vi "Main.vi"() -> ()   [LabVIEW 2017]
uses:
  Controls/SM_Control.ctl
  Controls/Operaciones.ctl
panel:
  in  "ON/OFF":bool
  in  "Clear":bool
  out "Display":string
  in  "Teclas":T1
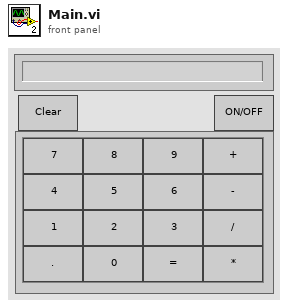
[diagram p1: front panel]
types:
  T1 = cluster{"Cero":bool, "Uno":bool, "Dos":bool, "Tres":bool, "Cuatro":bool, "Cinco":bool, "Seis":bool, "Siete":bool, "Ocho":bool, "Nueve":bool, "Punto":bool, "Igual":bool, "Mas":bool, "Resta":bool, "Div":bool, "Multp":bool}
  T2 = typedef "SM_Control.ctl" = enum16{"Inicializar", "Event Handler", "Tecla", "Stop", "Clear", "ON/OFF"}
  T3 = typedef "Operaciones.ctl" = enum16{"Suma", "Resta", "Mult", "Div"}
  T4 = enum8{"Enabled", "Disabled", "Disabled and Grayed Out"}
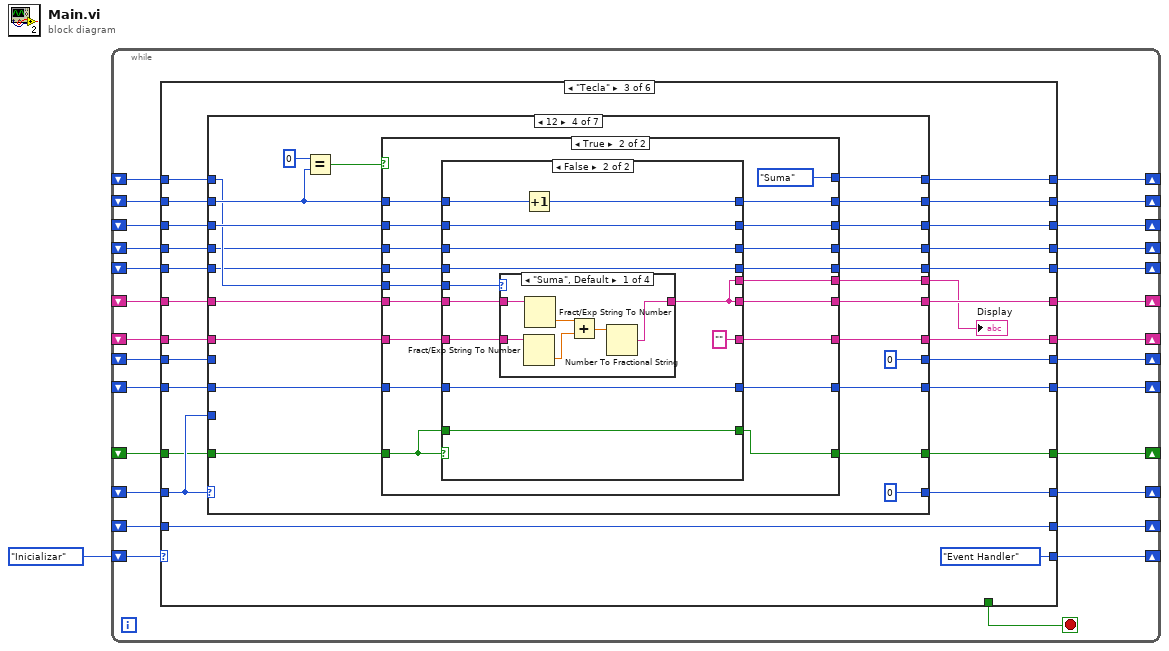
[diagram p0: block diagram]
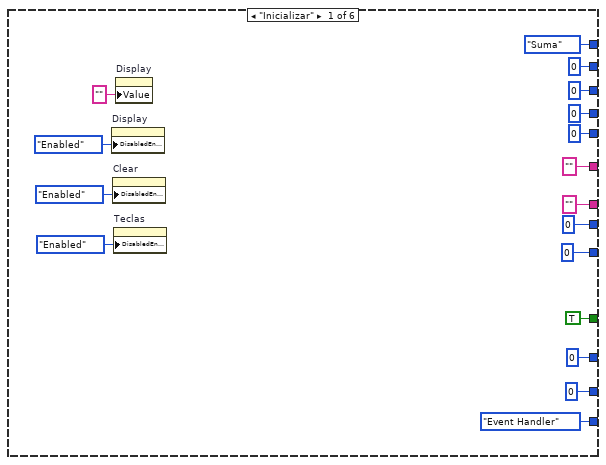
[diagram p2: hidden frame]
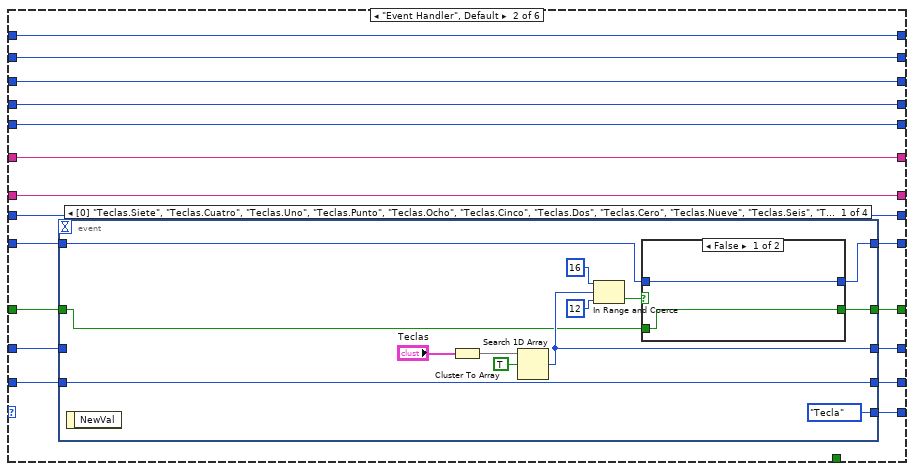
[diagram p3: hidden frame]
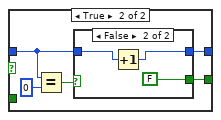
[diagram p4: hidden frame]
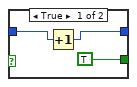
[diagram p5: hidden frame]
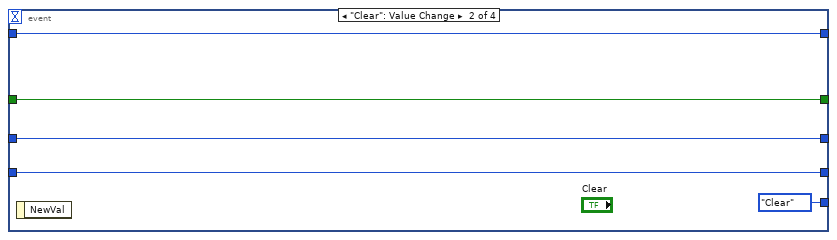
[diagram p6: hidden frame]
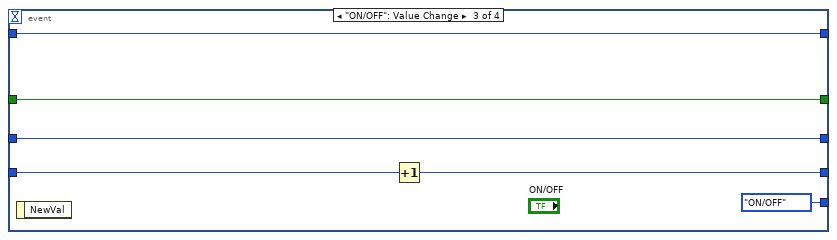
[diagram p7: hidden frame]
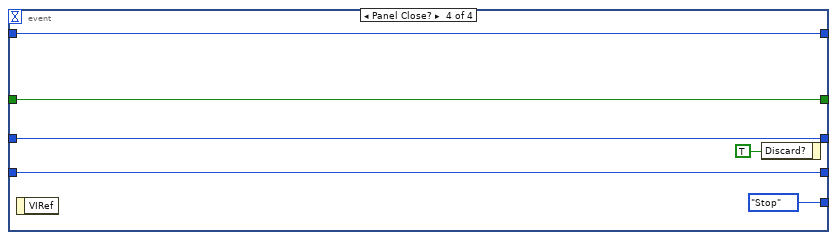
[diagram p8: hidden frame]
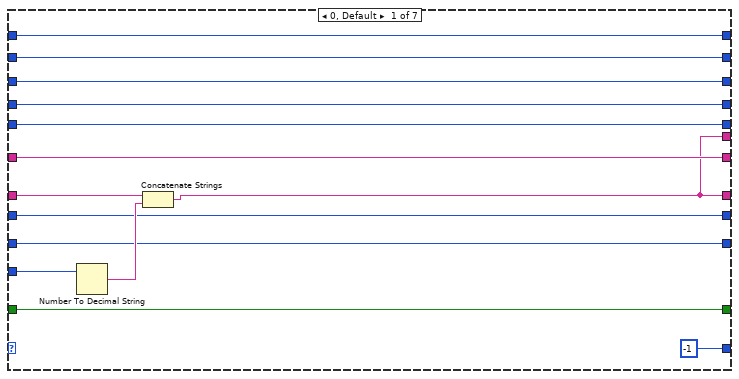
[diagram p9: hidden frame]
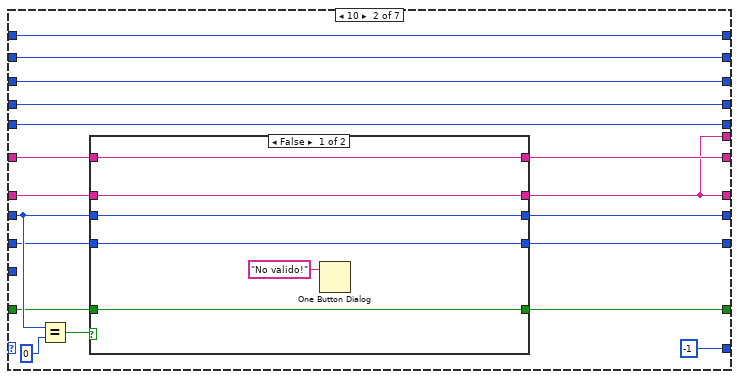
[diagram p10: hidden frame]
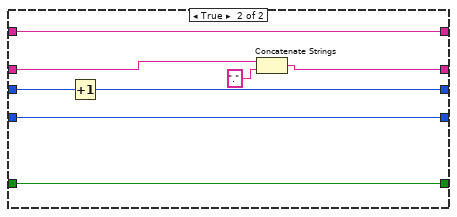
[diagram p11: hidden frame]
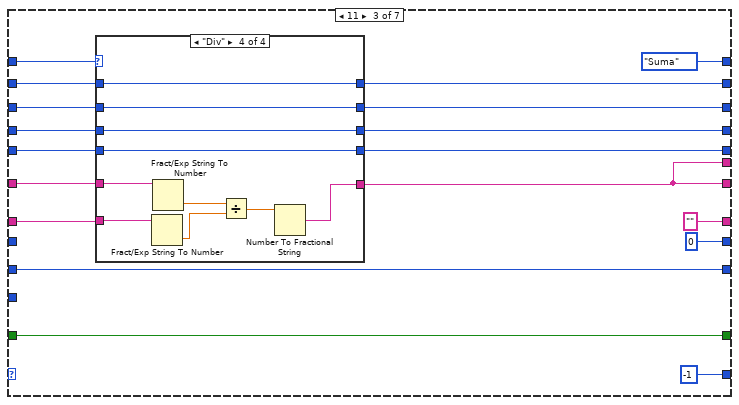
[diagram p12: hidden frame]
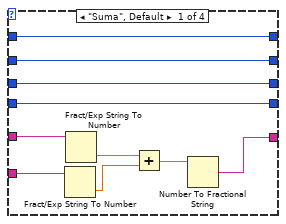
[diagram p13: hidden frame]
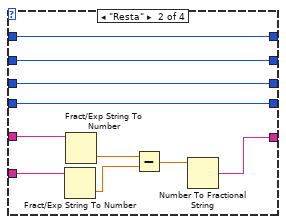
[diagram p14: hidden frame]
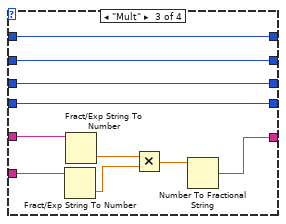
[diagram p15: hidden frame]
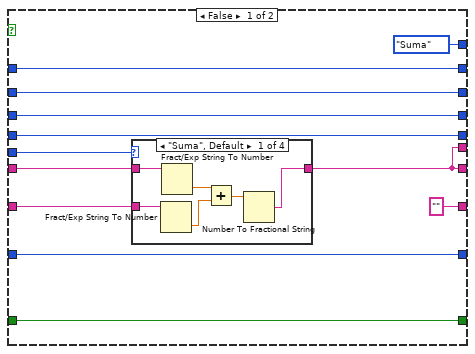
[diagram p16: hidden frame]
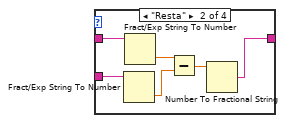
[diagram p17: hidden frame]
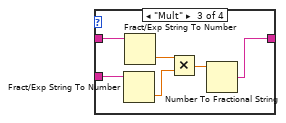
[diagram p18: hidden frame]
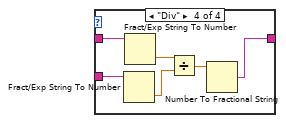
[diagram p19: hidden frame]
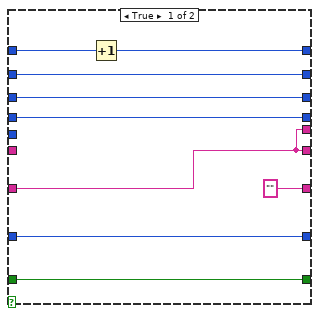
[diagram p20: hidden frame]
diagram:
  n1 = while {
    shift-right: [w27] -> _
    shift-left: SM_Control."Inicializar" -> [w28]
    shift-right: [w25] -> _
    shift-left: _ -> [w23]
    shift-right: [w24] -> _
    shift-left: _ -> [w22]
    shift-right: [w21] -> _
    shift-left: _ -> [w20]
    shift-right: [w19] -> _
    shift-left: _ -> [w18]
    shift-right: [w17] -> _
    shift-left: _ -> [w16]
    shift-right: [w15] -> _
    shift-left: _ -> [w14]
    shift-right: [w13] -> _
    shift-left: _ -> [w12]
    shift-right: [w11] -> _
    shift-left: _ -> [w10]
    shift-right: [w9] -> _
    shift-left: _ -> [w8]
    shift-right: [w7] -> _
    shift-left: _ -> [w6]
    shift-right: [w5] -> _
    shift-left: _ -> [w3]
    shift-right: [w4] -> _
    shift-left: _ -> [w2]
    stop <- w26 stop-if-true
    n2 = case shown="\"Tecla\"" w28 {
      tunnel: [SM_Control."Event Handler" w62 SM_Control."Event Handler" SM_Control."Inicializar" SM_Control."Event Handler" w769] -> w27
      tunnel: [_ _ _ TRUE _ _] -> w26
      tunnel: [0 ("index of element") w61 w128 w738 -1 ("index of element") w765] -> w25
      tunnel: [0 ("index of element") w58 w129 w737 w752 w768] -> w24
      tunnel: w23 -> [_ w60 w118 w738 _ w766]
      tunnel: w22 -> [_ w59 w129 w737 w752 w767]
      tunnel: ["" w57 w127 w736 "" w764] -> w21
      tunnel: w20 -> [_ w57 w126 w736 _ w764]
      tunnel: [0 ("index of element") w56 w124 w735 0 ("index of element") 0 ("index of element")] -> w19
      tunnel: w18 -> [_ w56 w125 w735 _ _]
      tunnel: ["" w55 w122 w734 "" w762] -> w17
      tunnel: w16 -> [_ w55 w123 w734 _ w762]
      tunnel: [Operaciones."Suma" w54 w121 w733 w748 w761] -> w15
      tunnel: w14 -> [_ w54 w120 w733 w748 w761]
      tunnel: [0 ("index of element") w53 w116 w732 0 ("index of element") w760] -> w13
      tunnel: w12 -> [_ w53 w117 w732 _ w760]
      tunnel: [0 ("index of element") w52 w114 w731 0 ("index of element") w759] -> w11
      tunnel: w10 -> [_ w52 w115 w731 _ w759]
      tunnel: [0 ("index of element") w48 w112 w730 0 ("index of element") w758] -> w9
      tunnel: w8 -> [_ w51 w113 w730 _ w758]
      tunnel: [TRUE w50 w110 w729 TRUE w757] -> w7
      tunnel: w6 -> [_ w49 w111 w729 _ w757]
      tunnel: [0 ("index of element") w47 w108 w728 0 ("index of element") w756] -> w5
      tunnel: [0 ("index of element") w46 w106 w727 0 ("index of element") w755] -> w4
      tunnel: w3 -> [_ w47 w109 w728 _ w756]
      tunnel: w2 -> [_ w46 w107 w727 _ w755]
      frame "Inicializar" {
        n3 = property on="Display" class="Str"("DisabledEnum"=T4."Enabled" ("Disabled")) -> ()  [unwired: 2 in, 2 out]
        n4 = property on="Clear" class="Bool"("DisabledEnum"=T4."Enabled" ("Disabled")) -> ()  [unwired: 2 in, 2 out]
        n5 = property on="Teclas" class="Clust"("DisabledEnum"=T4."Enabled" ("Disabled")) -> ()  [unwired: 2 in, 2 out]
        n6 = property on="Display" class="Str"("Value"="" ("Display")) -> ()  [unwired: 2 in, 2 out]
      }
      frame "Event Handler", Default {
        n7 = event shown="[0] \"Teclas.Siete\", \"Teclas.Cuatro\", \"Teclas.Uno\", \"Teclas.Punto\", \"Teclas.Ocho\", \"Teclas.Cinco\", \"Teclas.Dos\", \"Teclas.Cero\", \"Teclas.Nueve\", \"Teclas.Seis\", \"Teclas.Tres\", \"Teclas.Igual\", \"Teclas.Multp\", \"Teclas.Div\", \"Teclas.Resta\", \"Teclas.Mas\": Value Change" {
          selector: _ -> [_ _ _ _]
          dyn-events: _ -> [_ _ _ _]
          timeout: _ -> [_ _ _ _]
          tunnel: [SM_Control."Tecla" SM_Control."Clear" SM_Control."ON/OFF" SM_Control."Stop"] -> w62
          tunnel: [w70 w92 w98 w102] -> w61
          tunnel: w60 -> [_ w92 w98 w102]
          tunnel: [w71 w91 w96 w103] -> w58
          tunnel: w59 -> [w71 w91 w97 w103]
          tunnel: w51 -> [w66 w89 w95 w101]
          tunnel: [w65 w90 w94 w100] -> w50
          tunnel: w49 -> [w63 w90 w94 w100]
          tunnel: [w64 w89 w95 w101] -> w48
          event "Teclas.Siete", "Teclas.Cuatro", "Teclas.Uno", "Teclas.Punto", "Teclas.Ocho", "Teclas.Cinco", "Teclas.Dos", "Teclas.Cero", "Teclas.Nueve", "Teclas.Seis", "Teclas.Tres", "Teclas.Igual", "Teclas.Multp", "Teclas.Div", "Teclas.Resta", "Teclas.Mas": Value Change {
            n8 = event-data() -> ()  [unwired: 1 in, 1 out]
            n9 = Cluster To Array(cluster="Teclas") -> (array=w73:bool[])
            n10 = Search 1D Array(1D array=w73, element=TRUE) -> (index of element=w70:i32)  [unwired: 1 in]
            n11 = In Range and Coerce(upper limit=16, x=w70, lower limit=12) -> (In Range?=w67:bool)  [unwired: 1 out]
            n12 = case shown="False" w67 {
              tunnel: w66 -> [w77 w79]
              tunnel: [w76 w80] -> w65
              tunnel: [w77 w78] -> w64
              tunnel: w63 -> [w76 _]
              frame False {
              }
              frame True {
                n13 = Equal?(x=w79, y=0) -> (x = y?=w81:bool)
                n14 = case shown="False" w81 {
                  tunnel: [TRUE FALSE] -> w80
                  tunnel: w79 -> [w84 w87]
                  tunnel: [w83 w86] -> w78
                  frame True {
                    n15 = Increment(x=w84) -> (x+1=w83:i32)
                  }
                  frame False {
                    n16 = Increment(x=w87) -> (x+1=w86:i32)
                  }
                }
              }
            }
          }
          event "Clear": Value Change {
            n17 = event-data() -> ()  [unwired: 1 in, 1 out]
          }
          event "ON/OFF": Value Change {
            n18 = event-data() -> ()  [unwired: 1 in, 1 out]
            n19 = Increment(x=w97) -> (x+1=w96:i32)
          }
          event Panel Close? {
            n20 = event-data() -> ()  [unwired: 1 in, 1 out]
            n21 = event-data("Discard?"=TRUE) -> ()  [unwired: 1 in, 1 out]
          }
        }
      }
      frame "Tecla" {
        n22 = case shown="12" w118 {
          tunnel: [-1 ("index of element") -1 ("index of element") -1 ("index of element") 0 ("index of element") 0 ("index of element") 0 ("index of element") 0 ("index of element")] -> w128
          tunnel: [w139 w154 "" w244 w368 w491 w614] -> w127
          tunnel: w126 -> [w143 w162 w193 w257 w380 w503 w626]
          tunnel: w125 -> [w142 w159 _ _ _ _ _]
          tunnel: [w142 w158 0 ("index of element") 0 ("index of element") 0 ("index of element") 0 ("index of element") 0 ("index of element")] -> w124
          tunnel: [w141 w156 w189 w249 w373 w496 w619] -> w122
          tunnel: w123 -> [w141 w157 w194 w256 w379 w502 w625]
          tunnel: [w140 w155 Operaciones."Suma" w239 w363 w486 w609] -> w121
          tunnel: w120 -> [w140 w155 w192 w240 w364 w487 w610]
          tunnel: [w139 w154 w189 w248 w372 w495 w618] -> w119
          tunnel: w118 -> [w137 _ _ _ _ _ _]
          tunnel: [w136 w152 w185 w251 w375 w498 w621] -> w116
          tunnel: w117 -> [w136 w152 w186 w250 w374 w497 w620]
          tunnel: [w135 w151 w183 w252 w376 w499 w622] -> w114
          tunnel: w115 -> [w135 w151 w184 w253 w358 w482 w605]
          tunnel: w113 -> [w134 w150 w181 w242 w366 w489 w612]
          tunnel: [w134 w149 w181 w241 w365 w488 w611] -> w112
          tunnel: w111 -> [w133 w148 w182 w245 w369 w492 w615]
          tunnel: [w133 w147 w182 w243 w367 w490 w613] -> w110
          tunnel: w109 -> [w132 w146 w180 w238 w362 w481 w604]
          tunnel: [w132 w146 w179 w237 w361 w485 w608] -> w108
          tunnel: w107 -> [w131 w145 w178 w236 w360 w484 w607]
          tunnel: [w131 w145 w177 w235 w359 w483 w606] -> w106
          frame 0, Default {
            n23 = Number To Decimal String(number=w137) -> (decimal integer string=w144:string)  [unwired: 1 in]
            n24 = Concatenate Strings(w143, w144) -> (w139:string)
          }
          frame 10 {
            n25 = Equal?(x=w159, y=0) -> (x = y?=w161:bool)
            n26 = case shown="False" w161 {
              tunnel: w162 -> [w168 w175]
              tunnel: [w168 w174] -> w154
              tunnel: w159 -> [w167 w173]
              tunnel: [w167 w172] -> w158
              tunnel: w157 -> [w165 w171]
              tunnel: [w165 w171] -> w156
              tunnel: [w164 w170] -> w149
              tunnel: w150 -> [w164 w170]
              tunnel: w148 -> [w163 w169]
              tunnel: [w163 w169] -> w147
              frame False {
                n27 = One Button Dialog(message="No valido!") -> ()  [unwired: 1 in, 1 out]
              }
              frame True {
                n28 = Increment(x=w173) -> (x+1=w172:i32)
                n29 = Concatenate Strings(w175, "." ("string")) -> (w174:string)
              }
            }
          }
          frame 11 {
            n30 = case shown="\"Div\"" w192 {
              tunnel: w194 -> [w204 w214 w224 w234]
              tunnel: w193 -> [w203 w213 w223 w233]
              tunnel: [w199 w209 w219 w229] -> w189
              tunnel: [w198 w208 w218 w228] -> w185
              tunnel: w186 -> [w198 w208 w218 w228]
              tunnel: [w197 w207 w217 w227] -> w183
              tunnel: w184 -> [w197 w207 w217 w227]
              tunnel: [w196 w206 w216 w226] -> w179
              tunnel: w180 -> [w196 w206 w216 w226]
              tunnel: w178 -> [w195 w205 w215 w225]
              tunnel: [w195 w205 w215 w225] -> w177
              frame "Suma", Default {
                n31 = Fract/Exp String To Number(string=w203) -> (number=w201:dbl)  [unwired: 3 in, 1 out]
                n32 = Fract/Exp String To Number(string=w204) -> (number=w202:dbl)  [unwired: 3 in, 1 out]
                n33 = Add(x=w202, y=w201) -> (x+y=w200:dbl)
                n34 = Number To Fractional String(number=w200) -> (F-format string=w199:string)  [unwired: 3 in]
              }
              frame "Resta" {
                n35 = Fract/Exp String To Number(string=w213) -> (number=w211:dbl)  [unwired: 3 in, 1 out]
                n36 = Fract/Exp String To Number(string=w214) -> (number=w212:dbl)  [unwired: 3 in, 1 out]
                n37 = Subtract(x=w212, y=w211) -> (x-y=w210:dbl)
                n38 = Number To Fractional String(number=w210) -> (F-format string=w209:string)  [unwired: 3 in]
              }
              frame "Mult" {
                n39 = Fract/Exp String To Number(string=w223) -> (number=w221:dbl)  [unwired: 3 in, 1 out]
                n40 = Fract/Exp String To Number(string=w224) -> (number=w222:dbl)  [unwired: 3 in, 1 out]
                n41 = Multiply(x=w222, y=w221) -> (x*y=w220:dbl)
                n42 = Number To Fractional String(number=w220) -> (F-format string=w219:string)  [unwired: 3 in]
              }
              frame "Div" {
                n43 = Fract/Exp String To Number(string=w233) -> (number=w231:dbl)  [unwired: 3 in, 1 out]
                n44 = Fract/Exp String To Number(string=w234) -> (number=w232:dbl)  [unwired: 3 in, 1 out]
                n45 = Divide(x=w232, y=w231) -> (x/y=w230:dbl)
                n46 = Number To Fractional String(number=w230) -> (F-format string=w229:string)  [unwired: 3 in]
              }
            }
          }
          frame 12 {
            n47 = Equal?(x=0 ("y"), y=w250) -> (x = y?=w247:bool)
            n48 = case shown="True" w247 {
              tunnel: w257 -> [w262 w306]
              tunnel: w256 -> [w263 w308]
              tunnel: [w261 w307] -> w249
              tunnel: [w269 w309] -> w252
              tunnel: w253 -> [w269 w310]
              tunnel: w250 -> [w268 w312]
              tunnel: [w268 w311] -> w251
              tunnel: [w261 w305] -> w248
              tunnel: w245 -> [w266 w303]
              tunnel: ["" w304] -> w244
              tunnel: [w266 w302] -> w243
              tunnel: w242 -> [w265 w301]
              tunnel: [w265 w300] -> w241
              tunnel: w240 -> [w260 w299]
              tunnel: [Operaciones."Suma" Operaciones."Suma"] -> w239
              tunnel: w238 -> [w259 w297]
              tunnel: [w259 w296] -> w237
              tunnel: w236 -> [w258 w295]
              tunnel: [w258 w294] -> w235
              frame False {
                n49 = case shown="\"Suma\", Default" w260 {
                  tunnel: [w272 w278 w284 w290] -> w261
                  tunnel: w263 -> [w270 w277 w283 w289]
                  tunnel: w262 -> [w271 w276 w282 w288]
                  frame "Suma", Default {
                    n50 = Fract/Exp String To Number(string=w271) -> (number=w274:dbl)  [unwired: 3 in, 1 out]
                    n51 = Fract/Exp String To Number(string=w270) -> (number=w275:dbl)  [unwired: 3 in, 1 out]
                    n52 = Add(x=w275, y=w274) -> (x+y=w273:dbl)
                    n53 = Number To Fractional String(number=w273) -> (F-format string=w272:string)  [unwired: 3 in]
                  }
                  frame "Resta" {
                    n54 = Fract/Exp String To Number(string=w276) -> (number=w280:dbl)  [unwired: 3 in, 1 out]
                    n55 = Fract/Exp String To Number(string=w277) -> (number=w281:dbl)  [unwired: 3 in, 1 out]
                    n56 = Subtract(x=w281, y=w280) -> (x-y=w279:dbl)
                    n57 = Number To Fractional String(number=w279) -> (F-format string=w278:string)  [unwired: 3 in]
                  }
                  frame "Mult" {
                    n58 = Fract/Exp String To Number(string=w282) -> (number=w286:dbl)  [unwired: 3 in, 1 out]
                    n59 = Fract/Exp String To Number(string=w283) -> (number=w287:dbl)  [unwired: 3 in, 1 out]
                    n60 = Multiply(x=w287, y=w286) -> (x*y=w285:dbl)
                    n61 = Number To Fractional String(number=w285) -> (F-format string=w284:string)  [unwired: 3 in]
                  }
                  frame "Div" {
                    n62 = Fract/Exp String To Number(string=w288) -> (number=w292:dbl)  [unwired: 3 in, 1 out]
                    n63 = Fract/Exp String To Number(string=w289) -> (number=w293:dbl)  [unwired: 3 in, 1 out]
                    n64 = Divide(x=w293, y=w292) -> (x/y=w291:dbl)
                    n65 = Number To Fractional String(number=w291) -> (F-format string=w290:string)  [unwired: 3 in]
                  }
                }
              }
              frame True {
                n66 = case shown="False" w303 {
                  tunnel: w312 -> [w321 w333]
                  tunnel: [w320 w332] -> w311
                  tunnel: [w319 w331] -> w309
                  tunnel: w310 -> [w319 w331]
                  tunnel: w308 -> [_ w326]
                  tunnel: [w315 w325] -> w307
                  tunnel: w306 -> [w315 w327]
                  tunnel: [w315 w325] -> w305
                  tunnel: ["" ""] -> w304
                  tunnel: [w317 w330] -> w302
                  tunnel: w303 -> [w317 w330]
                  tunnel: [w316 w329] -> w300
                  tunnel: w301 -> [w316 w329]
                  tunnel: w299 -> [_ w328]
                  tunnel: [w314 w323] -> w296
                  tunnel: w297 -> [w314 w323]
                  tunnel: w295 -> [w313 w322]
                  tunnel: [w313 w322] -> w294
                  frame True {
                    n67 = Increment(x=w321) -> (x+1=w320:i32)
                  }
                  frame False {
                    n68 = case shown="\"Suma\", Default" w328 {
                      tunnel: w327 -> [w336 w342 w348 w354]
                      tunnel: w326 -> [w335 w341 w347 w353]
                      tunnel: [w334 w340 w346 w352] -> w325
                      frame "Suma", Default {
                        n69 = Fract/Exp String To Number(string=w336) -> (number=w338:dbl)  [unwired: 3 in, 1 out]
                        n70 = Fract/Exp String To Number(string=w335) -> (number=w339:dbl)  [unwired: 3 in, 1 out]
                        n71 = Add(x=w339, y=w338) -> (x+y=w337:dbl)
                        n72 = Number To Fractional String(number=w337) -> (F-format string=w334:string)  [unwired: 3 in]
                      }
                      frame "Resta" {
                        n73 = Fract/Exp String To Number(string=w342) -> (number=w344:dbl)  [unwired: 3 in, 1 out]
                        n74 = Fract/Exp String To Number(string=w341) -> (number=w345:dbl)  [unwired: 3 in, 1 out]
                        n75 = Subtract(x=w345, y=w344) -> (x-y=w343:dbl)
                        n76 = Number To Fractional String(number=w343) -> (F-format string=w340:string)  [unwired: 3 in]
                      }
                      frame "Mult" {
                        n77 = Fract/Exp String To Number(string=w348) -> (number=w350:dbl)  [unwired: 3 in, 1 out]
                        n78 = Fract/Exp String To Number(string=w347) -> (number=w351:dbl)  [unwired: 3 in, 1 out]
                        n79 = Multiply(x=w351, y=w350) -> (x*y=w349:dbl)
                        n80 = Number To Fractional String(number=w349) -> (F-format string=w346:string)  [unwired: 3 in]
                      }
                      frame "Div" {
                        n81 = Fract/Exp String To Number(string=w354) -> (number=w356:dbl)  [unwired: 3 in, 1 out]
                        n82 = Fract/Exp String To Number(string=w353) -> (number=w357:dbl)  [unwired: 3 in, 1 out]
                        n83 = Divide(x=w357, y=w356) -> (x/y=w355:dbl)
                        n84 = Number To Fractional String(number=w355) -> (F-format string=w352:string)  [unwired: 3 in]
                      }
                    }
                    n85 = Increment(x=w333) -> (x+1=w332:i32)
                  }
                }
              }
            }
          }
          frame 13 {
            n86 = Equal?(x=0 ("y"), y=w358) -> (x = y?=w371:bool)
            n87 = case shown="True" w371 {
              tunnel: w380 -> [w385 w429]
              tunnel: w379 -> [w386 w431]
              tunnel: [w384 w430] -> w373
              tunnel: [w392 w432] -> w376
              tunnel: w358 -> [w392 w433]
              tunnel: w374 -> [w391 w435]
              tunnel: [w391 w434] -> w375
              tunnel: [w384 w428] -> w372
              tunnel: w369 -> [w389 w426]
              tunnel: ["" w427] -> w368
              tunnel: [w389 w425] -> w367
              tunnel: w366 -> [w388 w424]
              tunnel: [w388 w423] -> w365
              tunnel: w364 -> [w383 w422]
              tunnel: [Operaciones."Resta" Operaciones."Resta"] -> w363
              tunnel: w362 -> [w382 w420]
              tunnel: [w382 w419] -> w361
              tunnel: w360 -> [w381 w418]
              tunnel: [w381 w417] -> w359
              frame False {
                n88 = case shown="\"Div\"" w383 {
                  tunnel: [w395 w401 w407 w413] -> w384
                  tunnel: w386 -> [w393 w400 w406 w412]
                  tunnel: w385 -> [w394 w399 w405 w411]
                  frame "Suma", Default {
                    n89 = Fract/Exp String To Number(string=w394) -> (number=w397:dbl)  [unwired: 3 in, 1 out]
                    n90 = Fract/Exp String To Number(string=w393) -> (number=w398:dbl)  [unwired: 3 in, 1 out]
                    n91 = Add(x=w398, y=w397) -> (x+y=w396:dbl)
                    n92 = Number To Fractional String(number=w396) -> (F-format string=w395:string)  [unwired: 3 in]
                  }
                  frame "Resta" {
                    n93 = Fract/Exp String To Number(string=w399) -> (number=w403:dbl)  [unwired: 3 in, 1 out]
                    n94 = Fract/Exp String To Number(string=w400) -> (number=w404:dbl)  [unwired: 3 in, 1 out]
                    n95 = Subtract(x=w404, y=w403) -> (x-y=w402:dbl)
                    n96 = Number To Fractional String(number=w402) -> (F-format string=w401:string)  [unwired: 3 in]
                  }
                  frame "Mult" {
                    n97 = Fract/Exp String To Number(string=w405) -> (number=w409:dbl)  [unwired: 3 in, 1 out]
                    n98 = Fract/Exp String To Number(string=w406) -> (number=w410:dbl)  [unwired: 3 in, 1 out]
                    n99 = Multiply(x=w410, y=w409) -> (x*y=w408:dbl)
                    n100 = Number To Fractional String(number=w408) -> (F-format string=w407:string)  [unwired: 3 in]
                  }
                  frame "Div" {
                    n101 = Fract/Exp String To Number(string=w411) -> (number=w415:dbl)  [unwired: 3 in, 1 out]
                    n102 = Fract/Exp String To Number(string=w412) -> (number=w416:dbl)  [unwired: 3 in, 1 out]
                    n103 = Divide(x=w416, y=w415) -> (x/y=w414:dbl)
                    n104 = Number To Fractional String(number=w414) -> (F-format string=w413:string)  [unwired: 3 in]
                  }
                }
              }
              frame True {
                n105 = case shown="False" w426 {
                  tunnel: w435 -> [w437 w446]
                  tunnel: [w437 w446] -> w434
                  tunnel: [w436 w445] -> w432
                  tunnel: w433 -> [w444 w456]
                  tunnel: w431 -> [_ w451]
                  tunnel: [w440 w450] -> w430
                  tunnel: w429 -> [w440 w452]
                  tunnel: [w440 w450] -> w428
                  tunnel: ["" ""] -> w427
                  tunnel: [w442 w455] -> w425
                  tunnel: w426 -> [w442 w455]
                  tunnel: [w441 w454] -> w423
                  tunnel: w424 -> [w441 w454]
                  tunnel: w422 -> [_ w453]
                  tunnel: [w439 w448] -> w419
                  tunnel: w420 -> [w439 w448]
                  tunnel: w418 -> [w438 w447]
                  tunnel: [w438 w447] -> w417
                  frame True {
                    n106 = Increment(x=w444) -> (x+1=w436:i32)
                  }
                  frame False {
                    n107 = case shown="\"Div\"" w453 {
                      tunnel: w452 -> [w459 w465 w471 w477]
                      tunnel: w451 -> [w458 w464 w470 w476]
                      tunnel: [w457 w463 w469 w475] -> w450
                      frame "Suma", Default {
                        n108 = Fract/Exp String To Number(string=w459) -> (number=w461:dbl)  [unwired: 3 in, 1 out]
                        n109 = Fract/Exp String To Number(string=w458) -> (number=w462:dbl)  [unwired: 3 in, 1 out]
                        n110 = Add(x=w462, y=w461) -> (x+y=w460:dbl)
                        n111 = Number To Fractional String(number=w460) -> (F-format string=w457:string)  [unwired: 3 in]
                      }
                      frame "Resta" {
                        n112 = Fract/Exp String To Number(string=w465) -> (number=w467:dbl)  [unwired: 3 in, 1 out]
                        n113 = Fract/Exp String To Number(string=w464) -> (number=w468:dbl)  [unwired: 3 in, 1 out]
                        n114 = Subtract(x=w468, y=w467) -> (x-y=w466:dbl)
                        n115 = Number To Fractional String(number=w466) -> (F-format string=w463:string)  [unwired: 3 in]
                      }
                      frame "Mult" {
                        n116 = Fract/Exp String To Number(string=w471) -> (number=w473:dbl)  [unwired: 3 in, 1 out]
                        n117 = Fract/Exp String To Number(string=w470) -> (number=w474:dbl)  [unwired: 3 in, 1 out]
                        n118 = Multiply(x=w474, y=w473) -> (x*y=w472:dbl)
                        n119 = Number To Fractional String(number=w472) -> (F-format string=w469:string)  [unwired: 3 in]
                      }
                      frame "Div" {
                        n120 = Fract/Exp String To Number(string=w477) -> (number=w479:dbl)  [unwired: 3 in, 1 out]
                        n121 = Fract/Exp String To Number(string=w476) -> (number=w480:dbl)  [unwired: 3 in, 1 out]
                        n122 = Divide(x=w480, y=w479) -> (x/y=w478:dbl)
                        n123 = Number To Fractional String(number=w478) -> (F-format string=w475:string)  [unwired: 3 in]
                      }
                    }
                    n124 = Increment(x=w456) -> (x+1=w445:i32)
                  }
                }
              }
            }
          }
          frame 14 {
            n125 = Equal?(x=0 ("y"), y=w481) -> (x = y?=w494:bool)
            n126 = case shown="True" w494 {
              tunnel: w503 -> [w508 w552]
              tunnel: w502 -> [w509 w554]
              tunnel: [w507 w553] -> w496
              tunnel: [w515 w555] -> w499
              tunnel: w482 -> [w515 w556]
              tunnel: w497 -> [w514 w558]
              tunnel: [w514 w557] -> w498
              tunnel: [w507 w551] -> w495
              tunnel: w492 -> [w512 w549]
              tunnel: ["" w550] -> w491
              tunnel: [w512 w548] -> w490
              tunnel: w489 -> [w511 w547]
              tunnel: [w511 w546] -> w488
              tunnel: w487 -> [w506 w545]
              tunnel: [Operaciones."Div" Operaciones."Div"] -> w486
              tunnel: w481 -> [w505 w543]
              tunnel: [w505 w542] -> w485
              tunnel: w484 -> [w504 w541]
              tunnel: [w504 w540] -> w483
              frame False {
                n127 = case shown="\"Div\"" w506 {
                  tunnel: [w518 w524 w530 w536] -> w507
                  tunnel: w509 -> [w516 w523 w529 w535]
                  tunnel: w508 -> [w517 w522 w528 w534]
                  frame "Suma", Default {
                    n128 = Fract/Exp String To Number(string=w517) -> (number=w520:dbl)  [unwired: 3 in, 1 out]
                    n129 = Fract/Exp String To Number(string=w516) -> (number=w521:dbl)  [unwired: 3 in, 1 out]
                    n130 = Add(x=w521, y=w520) -> (x+y=w519:dbl)
                    n131 = Number To Fractional String(number=w519) -> (F-format string=w518:string)  [unwired: 3 in]
                  }
                  frame "Resta" {
                    n132 = Fract/Exp String To Number(string=w522) -> (number=w526:dbl)  [unwired: 3 in, 1 out]
                    n133 = Fract/Exp String To Number(string=w523) -> (number=w527:dbl)  [unwired: 3 in, 1 out]
                    n134 = Subtract(x=w527, y=w526) -> (x-y=w525:dbl)
                    n135 = Number To Fractional String(number=w525) -> (F-format string=w524:string)  [unwired: 3 in]
                  }
                  frame "Mult" {
                    n136 = Fract/Exp String To Number(string=w528) -> (number=w532:dbl)  [unwired: 3 in, 1 out]
                    n137 = Fract/Exp String To Number(string=w529) -> (number=w533:dbl)  [unwired: 3 in, 1 out]
                    n138 = Multiply(x=w533, y=w532) -> (x*y=w531:dbl)
                    n139 = Number To Fractional String(number=w531) -> (F-format string=w530:string)  [unwired: 3 in]
                  }
                  frame "Div" {
                    n140 = Fract/Exp String To Number(string=w534) -> (number=w538:dbl)  [unwired: 3 in, 1 out]
                    n141 = Fract/Exp String To Number(string=w535) -> (number=w539:dbl)  [unwired: 3 in, 1 out]
                    n142 = Divide(x=w539, y=w538) -> (x/y=w537:dbl)
                    n143 = Number To Fractional String(number=w537) -> (F-format string=w536:string)  [unwired: 3 in]
                  }
                }
              }
              frame True {
                n144 = case shown="True" w549 {
                  tunnel: w558 -> [w561 w570]
                  tunnel: [w561 w570] -> w557
                  tunnel: [w560 w569] -> w555
                  tunnel: w556 -> [w560 w569]
                  tunnel: w554 -> [_ w575]
                  tunnel: [w564 w574] -> w553
                  tunnel: w552 -> [w564 w576]
                  tunnel: [w564 w574] -> w551
                  tunnel: ["" ""] -> w550
                  tunnel: [w566 w579] -> w548
                  tunnel: w549 -> [w566 w579]
                  tunnel: [w565 w578] -> w546
                  tunnel: w547 -> [w565 w578]
                  tunnel: w545 -> [_ w577]
                  tunnel: [w559 w568] -> w542
                  tunnel: w543 -> [w563 w572]
                  tunnel: w541 -> [w562 w571]
                  tunnel: [w562 w571] -> w540
                  frame True {
                    n145 = Increment(x=w563) -> (x+1=w559:i32)
                  }
                  frame False {
                    n146 = case shown="\"Div\"" w577 {
                      tunnel: w576 -> [w582 w588 w594 w600]
                      tunnel: w575 -> [w581 w587 w593 w599]
                      tunnel: [w580 w586 w592 w598] -> w574
                      frame "Suma", Default {
                        n147 = Fract/Exp String To Number(string=w582) -> (number=w584:dbl)  [unwired: 3 in, 1 out]
                        n148 = Fract/Exp String To Number(string=w581) -> (number=w585:dbl)  [unwired: 3 in, 1 out]
                        n149 = Add(x=w585, y=w584) -> (x+y=w583:dbl)
                        n150 = Number To Fractional String(number=w583) -> (F-format string=w580:string)  [unwired: 3 in]
                      }
                      frame "Resta" {
                        n151 = Fract/Exp String To Number(string=w588) -> (number=w590:dbl)  [unwired: 3 in, 1 out]
                        n152 = Fract/Exp String To Number(string=w587) -> (number=w591:dbl)  [unwired: 3 in, 1 out]
                        n153 = Subtract(x=w591, y=w590) -> (x-y=w589:dbl)
                        n154 = Number To Fractional String(number=w589) -> (F-format string=w586:string)  [unwired: 3 in]
                      }
                      frame "Mult" {
                        n155 = Fract/Exp String To Number(string=w594) -> (number=w596:dbl)  [unwired: 3 in, 1 out]
                        n156 = Fract/Exp String To Number(string=w593) -> (number=w597:dbl)  [unwired: 3 in, 1 out]
                        n157 = Multiply(x=w597, y=w596) -> (x*y=w595:dbl)
                        n158 = Number To Fractional String(number=w595) -> (F-format string=w592:string)  [unwired: 3 in]
                      }
                      frame "Div" {
                        n159 = Fract/Exp String To Number(string=w600) -> (number=w602:dbl)  [unwired: 3 in, 1 out]
                        n160 = Fract/Exp String To Number(string=w599) -> (number=w603:dbl)  [unwired: 3 in, 1 out]
                        n161 = Divide(x=w603, y=w602) -> (x/y=w601:dbl)
                        n162 = Number To Fractional String(number=w601) -> (F-format string=w598:string)  [unwired: 3 in]
                      }
                    }
                    n163 = Increment(x=w572) -> (x+1=w568:i32)
                  }
                }
              }
            }
          }
          frame 15 {
            n164 = Equal?(x=0 ("y"), y=w604) -> (x = y?=w617:bool)
            n165 = case shown="True" w617 {
              tunnel: w626 -> [w631 w675]
              tunnel: w625 -> [w632 w677]
              tunnel: [w630 w676] -> w619
              tunnel: [w638 w678] -> w622
              tunnel: w605 -> [w638 w679]
              tunnel: w620 -> [w637 w681]
              tunnel: [w637 w680] -> w621
              tunnel: [w630 w674] -> w618
              tunnel: w615 -> [w635 w672]
              tunnel: ["" w673] -> w614
              tunnel: [w635 w671] -> w613
              tunnel: w612 -> [w634 w670]
              tunnel: [w634 w669] -> w611
              tunnel: w610 -> [w629 w668]
              tunnel: [Operaciones."Mult" Operaciones."Mult"] -> w609
              tunnel: w604 -> [w628 w666]
              tunnel: [w628 w665] -> w608
              tunnel: w607 -> [w627 w664]
              tunnel: [w627 w663] -> w606
              frame False {
                n166 = case shown="\"Div\"" w629 {
                  tunnel: [w641 w647 w653 w659] -> w630
                  tunnel: w632 -> [w639 w646 w652 w658]
                  tunnel: w631 -> [w640 w645 w651 w657]
                  frame "Suma", Default {
                    n167 = Fract/Exp String To Number(string=w640) -> (number=w643:dbl)  [unwired: 3 in, 1 out]
                    n168 = Fract/Exp String To Number(string=w639) -> (number=w644:dbl)  [unwired: 3 in, 1 out]
                    n169 = Add(x=w644, y=w643) -> (x+y=w642:dbl)
                    n170 = Number To Fractional String(number=w642) -> (F-format string=w641:string)  [unwired: 3 in]
                  }
                  frame "Resta" {
                    n171 = Fract/Exp String To Number(string=w645) -> (number=w649:dbl)  [unwired: 3 in, 1 out]
                    n172 = Fract/Exp String To Number(string=w646) -> (number=w650:dbl)  [unwired: 3 in, 1 out]
                    n173 = Subtract(x=w650, y=w649) -> (x-y=w648:dbl)
                    n174 = Number To Fractional String(number=w648) -> (F-format string=w647:string)  [unwired: 3 in]
                  }
                  frame "Mult" {
                    n175 = Fract/Exp String To Number(string=w651) -> (number=w655:dbl)  [unwired: 3 in, 1 out]
                    n176 = Fract/Exp String To Number(string=w652) -> (number=w656:dbl)  [unwired: 3 in, 1 out]
                    n177 = Multiply(x=w656, y=w655) -> (x*y=w654:dbl)
                    n178 = Number To Fractional String(number=w654) -> (F-format string=w653:string)  [unwired: 3 in]
                  }
                  frame "Div" {
                    n179 = Fract/Exp String To Number(string=w657) -> (number=w661:dbl)  [unwired: 3 in, 1 out]
                    n180 = Fract/Exp String To Number(string=w658) -> (number=w662:dbl)  [unwired: 3 in, 1 out]
                    n181 = Divide(x=w662, y=w661) -> (x/y=w660:dbl)
                    n182 = Number To Fractional String(number=w660) -> (F-format string=w659:string)  [unwired: 3 in]
                  }
                }
              }
              frame True {
                n183 = case shown="False" w672 {
                  tunnel: w681 -> [w685 w694]
                  tunnel: [w685 w694] -> w680
                  tunnel: [w684 w693] -> w678
                  tunnel: w679 -> [w684 w693]
                  tunnel: w677 -> [_ w698]
                  tunnel: [w687 w697] -> w676
                  tunnel: w675 -> [w687 w699]
                  tunnel: [w687 w697] -> w674
                  tunnel: ["" ""] -> w673
                  tunnel: [w689 w702] -> w671
                  tunnel: w672 -> [w689 w702]
                  tunnel: [w688 w701] -> w669
                  tunnel: w670 -> [w688 w701]
                  tunnel: w668 -> [_ w700]
                  tunnel: [w683 w692] -> w665
                  tunnel: w666 -> [w683 w692]
                  tunnel: w664 -> [w686 w695]
                  tunnel: [w682 w691] -> w663
                  frame True {
                    n184 = Increment(x=w686) -> (x+1=w682:i32)
                  }
                  frame False {
                    n185 = Increment(x=w695) -> (x+1=w691:i32)
                    n186 = case shown="\"Suma\", Default" w700 {
                      tunnel: w699 -> [w705 w711 w717 w723]
                      tunnel: w698 -> [w704 w710 w716 w722]
                      tunnel: [w703 w709 w715 w721] -> w697
                      frame "Suma", Default {
                        n187 = Fract/Exp String To Number(string=w705) -> (number=w707:dbl)  [unwired: 3 in, 1 out]
                        n188 = Fract/Exp String To Number(string=w704) -> (number=w708:dbl)  [unwired: 3 in, 1 out]
                        n189 = Add(x=w708, y=w707) -> (x+y=w706:dbl)
                        n190 = Number To Fractional String(number=w706) -> (F-format string=w703:string)  [unwired: 3 in]
                      }
                      frame "Resta" {
                        n191 = Fract/Exp String To Number(string=w711) -> (number=w713:dbl)  [unwired: 3 in, 1 out]
                        n192 = Fract/Exp String To Number(string=w710) -> (number=w714:dbl)  [unwired: 3 in, 1 out]
                        n193 = Subtract(x=w714, y=w713) -> (x-y=w712:dbl)
                        n194 = Number To Fractional String(number=w712) -> (F-format string=w709:string)  [unwired: 3 in]
                      }
                      frame "Mult" {
                        n195 = Fract/Exp String To Number(string=w717) -> (number=w719:dbl)  [unwired: 3 in, 1 out]
                        n196 = Fract/Exp String To Number(string=w716) -> (number=w720:dbl)  [unwired: 3 in, 1 out]
                        n197 = Multiply(x=w720, y=w719) -> (x*y=w718:dbl)
                        n198 = Number To Fractional String(number=w718) -> (F-format string=w715:string)  [unwired: 3 in]
                      }
                      frame "Div" {
                        n199 = Fract/Exp String To Number(string=w723) -> (number=w725:dbl)  [unwired: 3 in, 1 out]
                        n200 = Fract/Exp String To Number(string=w722) -> (number=w726:dbl)  [unwired: 3 in, 1 out]
                        n201 = Divide(x=w726, y=w725) -> (x/y=w724:dbl)
                        n202 = Number To Fractional String(number=w724) -> (F-format string=w721:string)  [unwired: 3 in]
                      }
                    }
                  }
                }
              }
            }
          }
        }
        "Display" <- w119
      }
      frame "Stop" {
      }
      frame "Clear" {
        n203 = property on="Display" class="Str"("Value"="" ("Display")) -> ()  [unwired: 2 in, 2 out]
      }
      frame "ON/OFF" {
        n204 = Quotient & Remainder(x=w767, y=2) -> (x-y*floor(x/y)=w772:i32)  [unwired: 1 out]
        n205 = Equal?(x=w772, y=0) -> (x = y?=w770:bool)
        n206 = case shown="False" w770 {
          tunnel: [SM_Control."Event Handler" SM_Control."Clear"] -> w769
          tunnel: [w776 w782] -> w768
          tunnel: w767 -> [w776 w782]
          tunnel: w766 -> [w775 w781]
          tunnel: [w775 w781] -> w765
          frame True {
            n207 = property on="Clear" class="Bool"("DisabledEnum"=T4."Enabled" ("Disabled")) -> ()  [unwired: 2 in, 2 out]
            n208 = property on="Display" class="Str"("DisabledEnum"=T4."Enabled" ("Disabled")) -> ()  [unwired: 2 in, 2 out]
            n209 = property on="Teclas" class="Clust"("DisabledEnum"=T4."Enabled" ("Disabled")) -> ()  [unwired: 2 in, 2 out]
          }
          frame False {
            n210 = property on="Clear" class="Bool"("DisabledEnum"=T4."Disabled and Grayed Out" ("Disabled")) -> ()  [unwired: 2 in, 2 out]
            n211 = property on="Display" class="Str"("DisabledEnum"=T4."Disabled and Grayed Out" ("Disabled")) -> ()  [unwired: 2 in, 2 out]
            n212 = property on="Teclas" class="Clust"("DisabledEnum"=T4."Disabled and Grayed Out" ("Disabled")) -> ()  [unwired: 2 in, 2 out]
          }
        }
      }
    }
  }
